vi "NewErrorCode.vi"(8 "ErrorIn":errorcluster caption="Error In(no Error)", 11 "ReferenceIn":refnum<class "ErrorDefinitionSQLite.lvclass"> caption="Reference In") -> (0 "ErrorOut":errorcluster caption="Error Out", 2 "NewErrorCode":i32, 3 "ReferenceOut":refnum<class "ErrorDefinitionSQLite.lvclass"> caption="Reference Out")   [LabVIEW 2021, in "ErrorDefinitionSQLite.lvclass"]
uses:
  ErrorDefinitionSQLite.lvclass
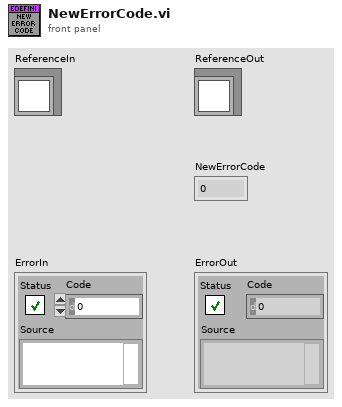
[diagram p1: front panel]
types:
  T1 = typedef "ErrorDefinitionSQLite.lvclass/ObjectAttributes.ctl" = cluster{"Path":path, "SQLiteRef":refnum<class "Connection.lvclass">, "EndOfRange":i32, "StartOfRange":i32}
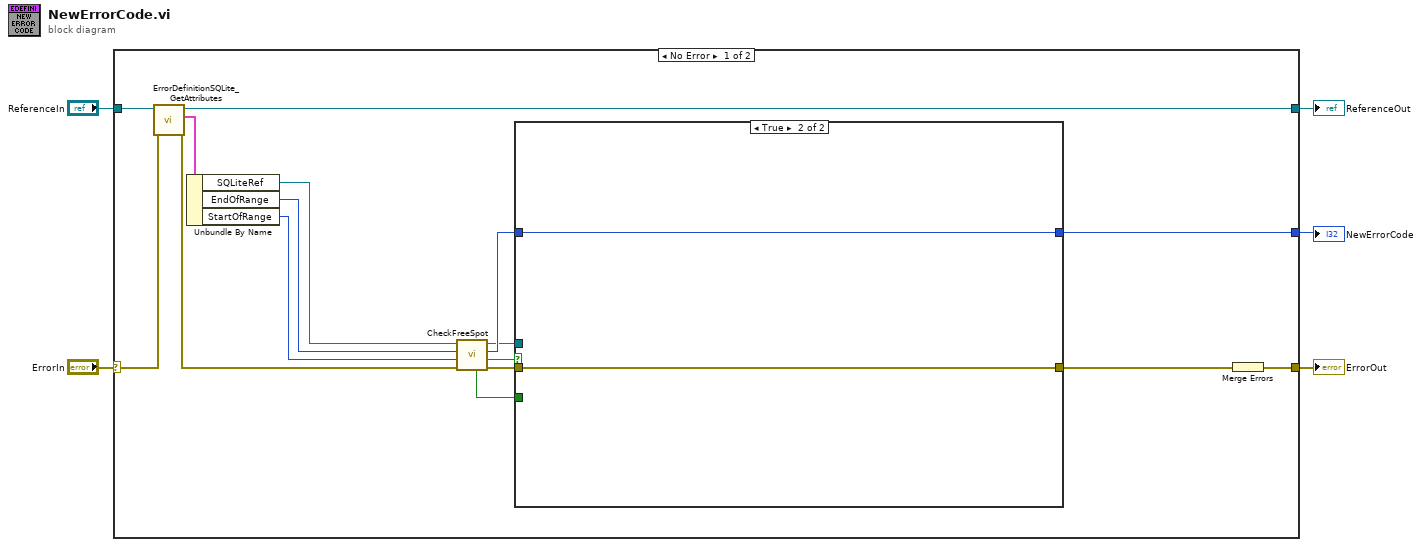
[diagram p0: block diagram]
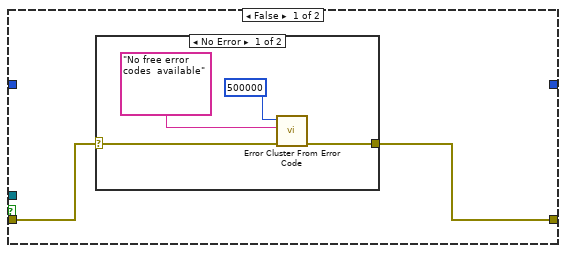
[diagram p2: hidden frame]
diagram:
  n1 = case shown="No Error" "ErrorIn" {
    selector: "ErrorIn" -> [w21 w32]
    tunnel: [w20 w32] -> w4
    tunnel: [w15 w31] -> w2
    tunnel: "ReferenceIn" -> [w16 w31]
    tunnel: [w11 _] -> w1
    frame No Error {
      n2 = call "ErrorDefinitionSQLite_GetAttributes.vi"("ErrorIn"=w21, "ReferenceIn"=w16) -> ("ErrorOut"=w18:errorcluster, "Data"=w14:T1, "ReferenceOut"=w15:refnum<class "ErrorDefinitionSQLite.lvclass">)  [unwired: 6 in, 1 out]
      n3 = Unbundle By Name(w14) -> ("SQLiteRef"=w8:refnum<class "Connection.lvclass">, "EndOfRange"=w7:i32, "StartOfRange"=w6:i32)
      n4 = call "CheckFreeSpot.vi"("ErrorIn"=w18, "MinError"=w6, "MaxError"=w7, "ConnectionIn"=w8) -> ("ErrorOut"=w19:errorcluster, "Valid"=w12:bool, "ErrorCode"=w13:i32, "ConnectionOut"=w9:refnum<class "Connection.lvclass">, "Existing"=w10:bool)  [unwired: 3 in]
      n5 = case shown="True" w12 {
        tunnel: [w22 w30] -> w17
        tunnel: w13 -> [_ w29]
        tunnel: w9 -> [_ _]
        tunnel: w19 -> [w23 w30]
        tunnel: [_ w29] -> w11
        tunnel: w10 -> [_ _]
        frame False {
          n6 = case shown="No Error" w23 {
            selector: w23 -> [w26 w28]
            tunnel: [w27 w28] -> w22
            frame No Error {
              n7 = call <vilib>:"Error Cluster From Error Code.vi"("error in (no error)"=w26, "error message (\"\")"="No free error codes  available" ("error message (\"\")"), "error code (0)"=500000) -> ("error out"=w27:errorcluster)  [unwired: 6 in]
            }
            frame Error {
            }
          }
        }
        frame True {
        }
      }
      n8 = Merge Errors(w17) -> (w20:errorcluster)
    }
    frame Error {
    }
  }
  "ErrorOut" <- w4
  "ReferenceOut" <- w2
  "NewErrorCode" <- w1
